vi "jkflipflop.vi"() -> ()   [LabVIEW 2020]
panel:
  in  "CLOCK":bool
  out "Q'":bool
  out "Q":bool
  in  "K":bool
  in  "J":bool
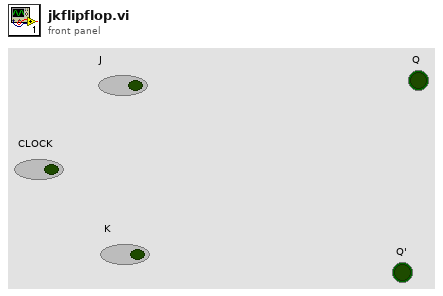
[diagram p1: front panel]
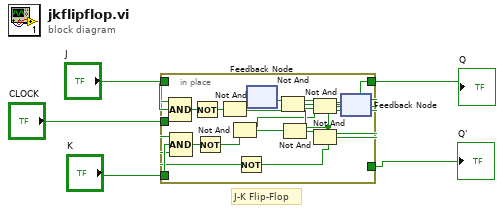
[diagram p0: block diagram]
diagram:
  # "J-K Flip-Flop"
  n1 = in-place {
    in-place-border: "J" -> [w16]
    in-place-border: "K" -> [w15]
    in-place-border: "CLOCK" -> [w13]
    in-place-border: [w11] -> w2
    in-place-border: [w10] -> w1
    n2 = Not(x=w13) -> (.not. x?=w14:bool)
    n3 = feedback #1() -> (w19:bool)  [unwired: 1 in]
    n4 = Not And(1:w14, 2:w19) -> (0:w18:bool)
    n5 = feedback #2() -> (w10:bool)  [unwired: 1 in]
    n6 = Compound Arithmetic op=AND(w13, w15, w10) -> (w7:bool)
    n7 = Not(x=w7) -> (.not. x?=w6:bool)
    n8 = Not And(1:w6, 2:w19) -> (0:w21:bool)
    n9 = Not And(1:w21, 2:w14) -> (0:w17:bool)
    n10 = Not And(1:w17, 2:w10) -> (0:w11:bool)
    n11 = Compound Arithmetic op=AND(w11, w16, w13) -> (w9:bool)
    n12 = Not(x=w9) -> (.not. x?=w8:bool)
    n13 = Not And(1:w21, 2:w8) -> (0:w20:bool)
    n14 = feedback-in #1(w20) -> ()
    n15 = Not And(1:w11, 2:w18) -> (0:w12:bool)
    n16 = feedback-in #2(w12) -> ()
  }
  "Q" <- w1
  "Q'" <- w2
